vi "SwerveDriveKinematics_Example.vi"() -> ()   [LabVIEW 2019]
uses:
  <vilib>/Rock Robotics/WPI/ThirdParty/JAS_Junk/TrajLib/TypeDef/CHASSIS_SPEEDS.ctl
  <vilib>/Rock Robotics/WPI/ThirdParty/JAS_Junk/TrajLib/Conv_Deg_Radians.vi
  <vilib>/Rock Robotics/WPI/ThirdParty/JAS_Junk/TrajLib/Rotation2d_CreateAngle.vi
  <vilib>/Rock Robotics/WPI/ThirdParty/JAS_Junk/TrajLib/Trajectory_Library.lvlib
panel:
  out "Rear Right Degrees":dbl format="%14.1f"
  out "Rear Left Degrees":dbl format="%14.1f"
  out "Front Right Degrees":dbl format="%14.1f"
  out "Front Left Degrees":dbl format="%14.1f"
  in  "Rear Right Angle \nDegrees":dbl format="%#_13g"
  in  "Rear Left Angle \nDegrees":dbl format="%#_13g"
  in  "Front Right Angle \nDegrees":dbl format="%#_13g"
  in  "Front Left Angle \nDegrees":dbl format="%#_13g"
  out "Rear Right\nVelocity Ft/Sec":dbl format="%13.2f"
  out "Rear Left\nVelocity Ft/Sec":dbl format="%13.2f"
  in  "Rear Right \nWheel Velocity\nFt/Sec":dbl
  in  "Rear Left \nWheel Velocity\nFT/Sec":dbl
  out "Front Right\nVelocity Ft/Sec":dbl format="%13.2f"
  out "Front Left\nVelocity Ft/Sec":dbl format="%13.2f"
  out "CHASSIS Speed\nM/S":T1 {"vOmega" format="%10.3f"; "vY" format="%10.3f"; "vX" format="%10.3f"}
  in  "Step":bool
  in  "Front Right \nWheel Velocity\nFt/Sec":dbl
  in  "Front Left \nWheel Velocity\nFT/Sec":dbl
  # "Swerve Drive Kinematics Example"
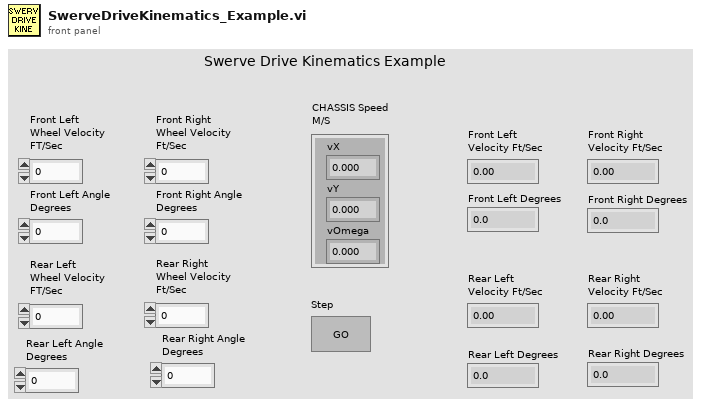
[diagram p1: front panel]
types:
  T1 = typedef "Trajectory_Library.lvlib/CHASSIS_SPEEDS.ctl" = cluster{"vX":dbl, "vY":dbl, "vOmega":dbl}
  T2 = typedef "Trajectory_Library.lvlib/TRANSLATION2D.ctl" = cluster{"X":dbl, "Y":dbl}
  T3 = typedef "Trajectory_Library.lvlib/SWERVE_DRIVE_KINEMATICS.ctl" = cluster{"NumModules":i32, "InverseKinematics":T4, "ForwardKinematics":T4, "Modules":T2[], "PrevCoR":T2, "SavedModuleStates":T5[]}
  T4 = typedef "NI_Matrix.lvlib/RealMatrix.ctl" = dbl[][]
  T5 = typedef "Trajectory_Library.lvlib/SWERVE_DRIVE_MODULE_STATE.ctl" = cluster{"Speed":dbl, "Angle":T6}
  T6 = typedef "Trajectory_Library.lvlib/ROTATION2D.ctl" = cluster{"VALUE":dbl, "COS":dbl, "SIN":dbl}
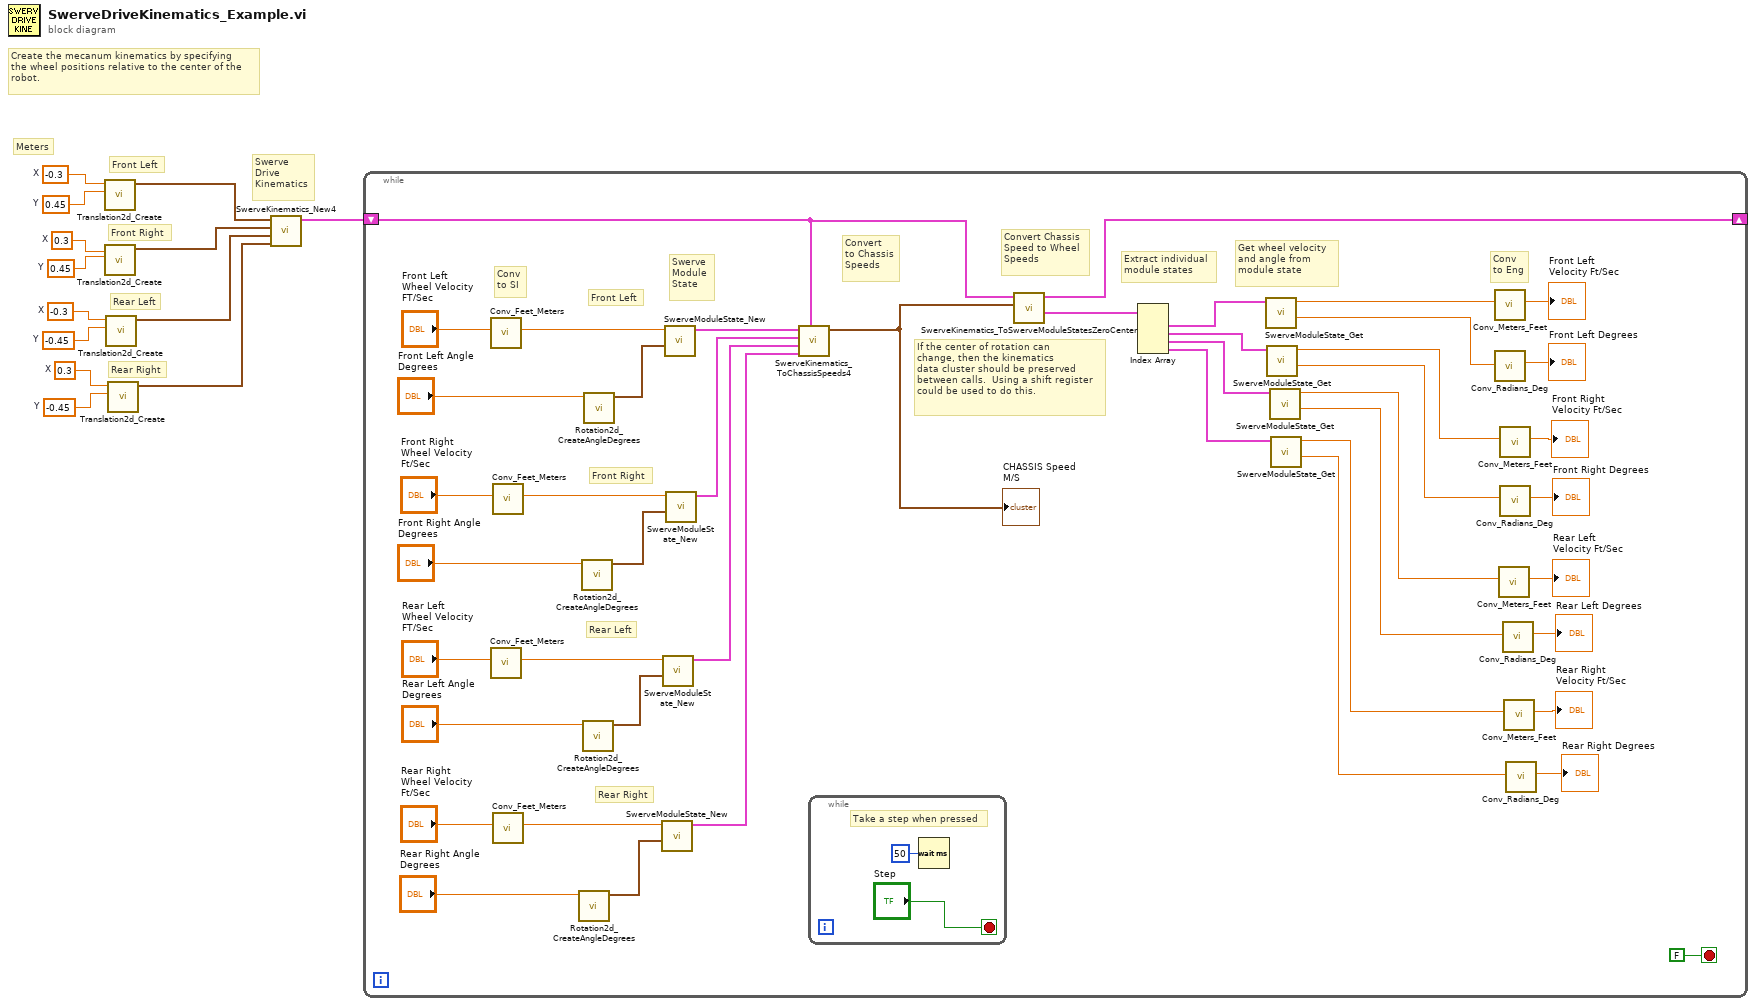
[diagram p0: block diagram]
diagram:
  w6 = -0.3  # X
  w7 = 0.45  # Y
  w8 = 0.3  # X
  w9 = 0.45  # Y
  w10 = -0.3  # X
  w11 = -0.45  # Y
  w12 = 0.3  # X
  w13 = -0.45  # Y
  # "Meters"
  # "Rear Right"
  # "Rear Left"
  # "Front Right"
  # "Front Left"
  # "Create the mecanum kinematics by specifying\nthe wheel positions relative to the center of the\nrobot."
  # "Swerve\nDrive\nKinematics"
  n1 = call <vilib>:"Translation2d_Create.vi"("Y"=w7, "X"=w6) -> ("TRANSLATION"=w5:T2)  [unwired: 9 in]
  n2 = call <vilib>:"Translation2d_Create.vi"("Y"=w9, "X"=w8) -> ("TRANSLATION"=w4:T2)  [unwired: 9 in]
  n3 = call <vilib>:"Translation2d_Create.vi"("Y"=w11, "X"=w10) -> ("TRANSLATION"=w3:T2)  [unwired: 9 in]
  n4 = call <vilib>:"Translation2d_Create.vi"("Y"=w13, "X"=w12) -> ("TRANSLATION"=w2:T2)  [unwired: 9 in]
  n5 = call <vilib>:"SwerveKinematics_New4.vi"("wheel 3"=w2, "wheel 2"=w3, "wheel 1"=w4, "wheel 0"=w5) -> ("SWERVE_DRIVE_KINEMATICS"=w1:T3)  [unwired: 7 in]
  n6 = while {
    shift-right: [w31] -> _
    shift-left: w1 -> [w49]
    stop <- FALSE stop-if-true
    # "Get wheel velocity \nand angle from \nmodule state"
    # "Front Left"
    # "Swerve\nModule\nState"
    # "Rear Right"
    # "Rear Left"
    # "Front Right"
    # "If the center of rotation can\nchange, then the kinematics\ndata cluster should be preserved\nbetween calls.  Using a shift register\ncould be used to do this."
    # "Extract individual\nmodule states"
    # "Conv\nto Eng"
    # "Conv\nto SI"
    # "Convert Chassis\nSpeed to Wheel\nSpeeds"
    # "Convert\nto Chassis\nSpeeds"
    n7 = call <vilib>:"Conv_Feet_Meters.vi"("Feet"="Front Left \nWheel Velocity\nFT/Sec") -> ("Meters"=w39:dbl)  [unwired: 10 in]
    n8 = call <vilib>:"Conv_Feet_Meters.vi"("Feet"="Rear Left \nWheel Velocity\nFT/Sec") -> ("Meters"=w37:dbl)  [unwired: 10 in]
    n9 = call <vilib>:"Conv_Feet_Meters.vi"("Feet"="Front Right \nWheel Velocity\nFt/Sec") -> ("Meters"=w38:dbl)  [unwired: 10 in]
    n10 = call <vilib>:"Conv_Feet_Meters.vi"("Feet"="Rear Right \nWheel Velocity\nFt/Sec") -> ("Meters"=w36:dbl)  [unwired: 10 in]
    n11 = call <vilib>:"Rotation2d_CreateAngleDegrees.vi"("Angle_Degrees"="Rear Right Angle \nDegrees") -> ("ROTATION"=w44:T6)  [unwired: 10 in]
    n12 = call <vilib>:"Rotation2d_CreateAngleDegrees.vi"("Angle_Degrees"="Front Right Angle \nDegrees") -> ("ROTATION"=w46:T6)  [unwired: 10 in]
    n13 = call <vilib>:"Rotation2d_CreateAngleDegrees.vi"("Angle_Degrees"="Rear Left Angle \nDegrees") -> ("ROTATION"=w45:T6)  [unwired: 10 in]
    n14 = call <vilib>:"Rotation2d_CreateAngleDegrees.vi"("Angle_Degrees"="Front Left Angle \nDegrees") -> ("ROTATION"=w47:T6)  [unwired: 10 in]
    n15 = call <vilib>:"SwerveModuleState_New.vi"("ROTATION"=w44, "Speed"=w36) -> ("SWERVE_DRIVE_MODULE_STATE"=w32:T5)  [unwired: 9 in]
    n16 = call <vilib>:"SwerveModuleState_New.vi"("ROTATION"=w45, "Speed"=w37) -> ("SWERVE_DRIVE_MODULE_STATE"=w33:T5)  [unwired: 9 in]
    n17 = call <vilib>:"SwerveModuleState_New.vi"("ROTATION"=w47, "Speed"=w39) -> ("SWERVE_DRIVE_MODULE_STATE"=w35:T5)  [unwired: 9 in]
    n18 = call <vilib>:"SwerveModuleState_New.vi"("ROTATION"=w46, "Speed"=w38) -> ("SWERVE_DRIVE_MODULE_STATE"=w34:T5)  [unwired: 9 in]
    n19 = call <vilib>:"SwerveKinematics_ToChassisSpeeds4.vi"("in SWERVE_DRIVE_KINEMATICS"=w49, "Wheel State 3"=w32, "Wheel State 2"=w33, "Wheel State 1"=w34, "Wheel State 0"=w35) -> ("Chassis Speed"=w48:T1)  [unwired: 6 in]
    "CHASSIS Speed\nM/S" <- w48
    n20 = while {
      stop <- "Step" stop-if-true
      # "Take a step when pressed"
      n21 = Wait (ms)(milliseconds to wait=u32 50) -> ()  [unwired: 1 out]
    }
    n22 = call <vilib>:"SwerveKinematics_ToSwerveModuleStatesZeroCenter.vi"("ChassisSpeeds"=w48, "in SWERVE_DRIVE_KINEMATICS"=w49) -> ("ModuleStates"=w30:T5[], "out SWERVE_DRIVE_KINEMATICS"=w31:T3)  [unwired: 8 in]
    n23 = Index Array(array=w30) -> (element #1=w29:T5, element #2=w28:T5, element #3=w27:T5, element #4=w26:T5)  [unwired: 4 in]
    n24 = call <vilib>:"SwerveModuleState_Get.vi"("Desired State"=w29) -> ("Angle RADIANS"=w22:dbl, "Speed M/S"=w25:dbl)  [unwired: 9 in]
    n25 = call <vilib>:"SwerveModuleState_Get.vi"("Desired State"=w28) -> ("Angle RADIANS"=w21:dbl, "Speed M/S"=w24:dbl)  [unwired: 9 in]
    n26 = call <vilib>:"SwerveModuleState_Get.vi"("Desired State"=w27) -> ("Angle RADIANS"=w19:dbl, "Speed M/S"=w20:dbl)  [unwired: 9 in]
    n27 = call <vilib>:"SwerveModuleState_Get.vi"("Desired State"=w26) -> ("Angle RADIANS"=w18:dbl, "Speed M/S"=w23:dbl)  [unwired: 9 in]
    n28 = call <vilib>:"Conv_Meters_Feet.vi"("Meters"=w25) -> ("Feet"=→"Front Left\nVelocity Ft/Sec":dbl)  [unwired: 10 in]
    n29 = call <vilib>:"Conv_Radians_Deg.vi"("Radians"=w22) -> ("Degrees"=→"Front Left Degrees":dbl)  [unwired: 10 in]
    n30 = call <vilib>:"Conv_Meters_Feet.vi"("Meters"=w20) -> ("Feet"=→"Rear Left\nVelocity Ft/Sec":dbl)  [unwired: 10 in]
    n31 = call <vilib>:"Conv_Meters_Feet.vi"("Meters"=w24) -> ("Feet"=→"Front Right\nVelocity Ft/Sec":dbl)  [unwired: 10 in]
    n32 = call <vilib>:"Conv_Radians_Deg.vi"("Radians"=w21) -> ("Degrees"=→"Front Right Degrees":dbl)  [unwired: 10 in]
    n33 = call <vilib>:"Conv_Radians_Deg.vi"("Radians"=w19) -> ("Degrees"=→"Rear Left Degrees":dbl)  [unwired: 10 in]
    n34 = call <vilib>:"Conv_Meters_Feet.vi"("Meters"=w23) -> ("Feet"=→"Rear Right\nVelocity Ft/Sec":dbl)  [unwired: 10 in]
    n35 = call <vilib>:"Conv_Radians_Deg.vi"("Radians"=w18) -> ("Degrees"=→"Rear Right Degrees":dbl)  [unwired: 10 in]
  }
